vi "Sel Measure_Bio_Type.vi"(8 "error in (no error)":errorcluster caption="错误输入（无错误）", 9 "condition":string, 11 "connection reference":T2) -> (0 "error out":errorcluster caption="错误输出", 2 "Measure_Bio_Typea":T1[](array[typedef]))   [LabVIEW 2015, in "Database Processing.lvlib"]
doc: "该模板用于创建子VI。"
uses:
  Database Processing.lvlib
  <vilib>/addons/database/Connection.llb/Conn ObjectReference.ctl
  Support/Table/Measure_Bio_Type.ctl
  <vilib>/addons/database/_DB Variant To Data/Database Variant To Data.xnode
  <vilib>/addons/database/NI_Database_API.lvlib
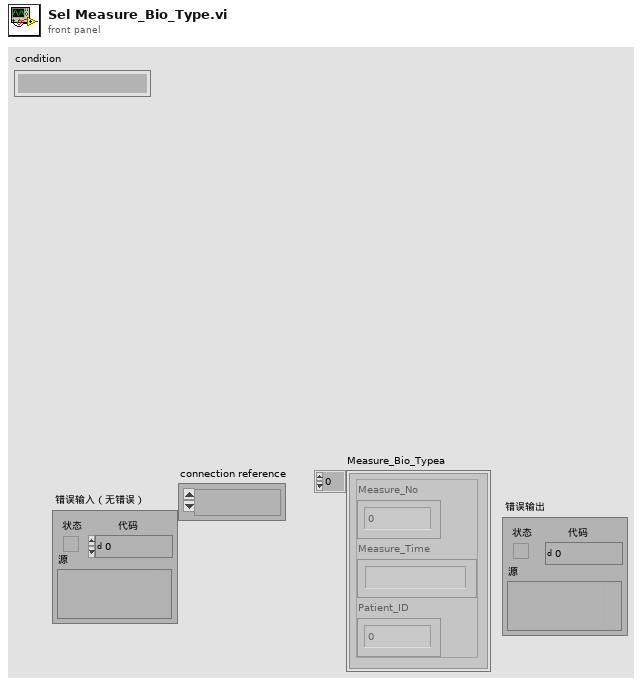
[diagram p1: front panel]
types:
  T1 = typedef "Database Processing.lvlib/Measure_Bio_Type.ctl" = cluster{"Measure_No":i64, "Measure_Time":string, "Patient_ID":i64}
  T2 = typedef "NI_Database_API.lvlib/Conn ObjectReference.ctl" = refnum<k1>
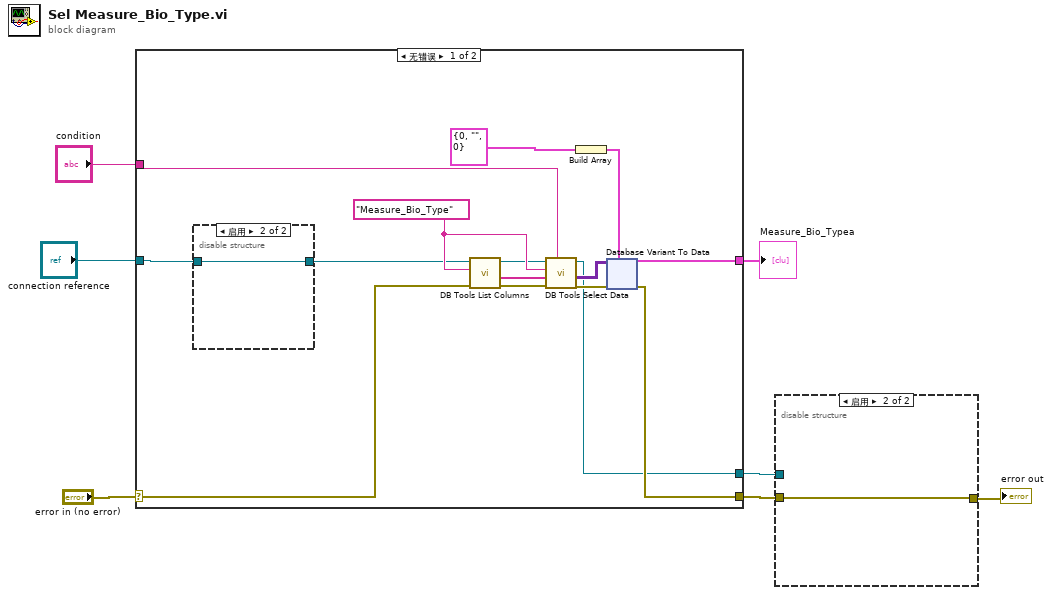
[diagram p0: block diagram]
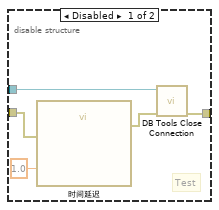
[diagram p2: hidden frame]
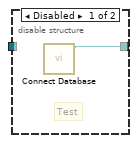
[diagram p3: hidden frame]
diagram:
  n1 = case shown="无错误" "error in (no error)" {
    selector: "error in (no error)" -> [w21 w128]
    tunnel: [w17 w128] -> w3
    tunnel: "connection reference" -> [w12 w127]
    tunnel: [w16 _] -> w5
    tunnel: "condition" -> [w13 _]
    tunnel: [w8 w127] -> w1
    frame No Error {
      w14 = "Measure_Bio_Type" ("table")
      n2 = disable-structure shown="启用" {
        disable-tunnel: [w22 w23] -> w9
        disable-tunnel: w12 -> [_ w23]
        frame Disabled {
          # "Test"
          n3 = call "Connect Database.vi"() -> ("connection reference"=w22:T2)  [unwired: 10 in, 1 out]
        }
        frame Enabled {
        }
      }
      n4 = call <vilib>:"DB Tools List Columns.vi"("table"=w14, "connection reference"=w9) -> ("columns"=w15:string[], "connection reference out"=w10:T2)  [unwired: 2 in, 2 out]
      n5 = call <vilib>:"DB Tools Select Data.vi"("condition"=w13, "error in (no error)"=w21, "columns"=w15, "table"=w14, "connection reference"=w10) -> ("error out"=w20:errorcluster, "data"=w19:variant[][], "connection reference out"=w8:T2)  [unwired: 1 in]
      n6 = Build Array(T1 {"Measure_No"=0, "Measure_Time"="", "Patient_ID"=0} ("Measure_Bio_Type")) -> (w18:T1[])
      n7 = xnode "Database Variant To Data"("database variant"=w19, "error in (no error)"=w20, "type"=w18) -> ("data"=w16:T1[], "error out"=w17:errorcluster)
    }
    frame Error {
    }
  }
  "Measure_Bio_Typea" <- w5
  n8 = disable-structure shown="启用" {
    disable-tunnel: w3 -> [w131 w134]
    disable-tunnel: [w133 w134] -> w2
    disable-tunnel: w1 -> [w132 _]
    frame Disabled {
      # "Test"
      n9 = call "时间延迟"("error in (no error)"=w131, "Delay Time (s)"=1.0) -> ("error out"=w130:errorcluster)  [unwired: 9 in]
      n10 = call <vilib>:"DB Tools Close Connection.vi"("error in (no error)"=w130, "connection reference"=w132) -> ("error out"=w133:errorcluster)  [unwired: 5 in]
    }
    frame Enabled {
    }
  }
  "error out" <- w2
